vi "Adjust_VI_Properties.vi"(6 "VI refnum in":refnum<vi>, 8 "error in (no error)":errorcluster, 9 "sourceInclusion":T3, 10 "properties in":T1[](array[typedef]), 11 "AB_EXE in":refnum<class "AB_EXE.lvclass">) -> (0 "error out":errorcluster, 1 "defaultSaveLevel":u32, 2 "properties out":T1[](array[typedef]), 3 "AB_EXE out":refnum<class "AB_EXE.lvclass">)   [LabVIEW 2020, in "AB_EXE.lvclass"]
uses:
  <vilib>/AppBuilder/AB_Classes/EXE/AB_EXE.lvclass
  <vilib>/AppBuilder/AB_Source_Inclusion.ctl
  <vilib>/AppBuilder/AB_Source_Properties.ctl
  <vilib>/AppBuilder/AB_Source_Property_Type.ctl
  <vilib>/AppBuilder/AB_Classes/Application/AB_Application.lvclass
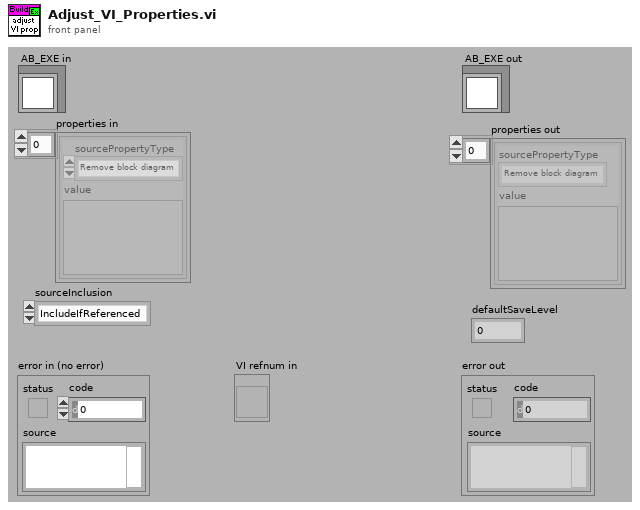
[diagram p1: front panel]
types:
  T1 = typedef "AB_Source_Properties.ctl" = cluster{"sourcePropertyType":T2, "value":variant}
  T2 = typedef "AB_Source_Property_Type.ctl" = enum16{"Remove block diagram", "Remove front panel", "Password", "Window has title bar", "Show menu bar", "Show vertical scroll bar", "Show horizontal scroll bar", "Show toolbar", "Show Abort button", "Show fp when called", "Window behavior", "Allow user to close window", "Window run-time position", "Run when opened", "Allow debugging", "Auto error handling", "Generate guard code", "Use stack variables", "Expression folding", "Integer only", "Inline subVI"}
  T3 = typedef "AB_Source_Inclusion.ctl" = enum16{"IncludeIfReferenced", "Include", "Exclude", "TopLevel"}
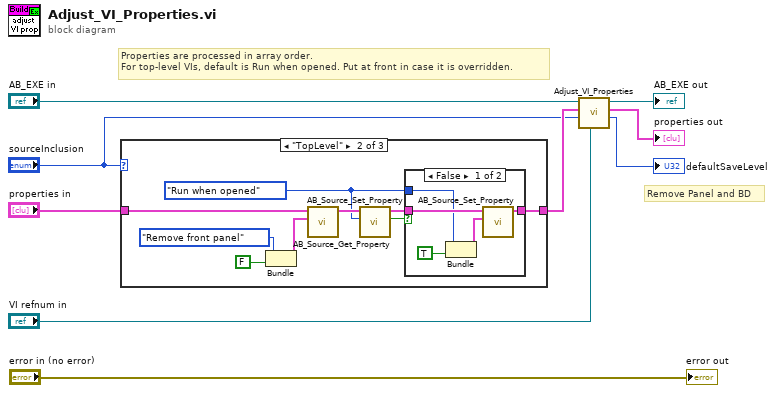
[diagram p0: block diagram]
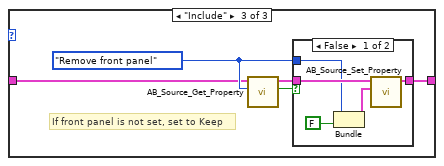
[diagram p4: hidden frame]
diagram:
  # "Remove Panel and BD"
  # "Properties are processed in array order.\nFor top-level VIs, default is Run when opened. Put at front in case it is overridden."
  n1 = case shown="\"TopLevel\"" "sourceInclusion" {
    tunnel: "properties in" -> [w10 w17 w26]
    tunnel: [w10 w12 w28] -> w3
    frame Default {
    }
    frame "TopLevel" {
      w11 = AB_Source_Property_Type."Run when opened" ("sourcePropertyType")
      n2 = Bundle("sourcePropertyType"=AB_Source_Property_Type."Remove front panel", FALSE) -> (w16:cluster{"sourcePropertyType":T2, bool})  [unwired: 1 out]
      n3 = call <vilib>:"AB_Source_Set_Property.vi"("sourceProperty"=w16, "sourceProperties in"=w17) -> ("sourceProperties out"=w15:T1[])  [unwired: 1 in, 8 out]
      n4 = call <vilib>:"AB_Source_Get_Property.vi"("type"=w11, "sourceProperties in"=w15) -> ("found"=w14:bool, "sourceProperties out"=w13:T1[])  [unwired: 1 in, 7 out]
      n5 = case shown="False" w14 {
        tunnel: w13 -> [w24 w25]
        tunnel: [w23 w25] -> w12
        tunnel: w11 -> [w21 _]
        frame False {
          n6 = Bundle("sourcePropertyType"=w21, TRUE) -> (w20:cluster{"sourcePropertyType":T2, bool})  [unwired: 1 out]
          n7 = call <vilib>:"AB_Source_Set_Property.vi"("sourceProperty"=w20, "sourceProperties in"=w24) -> ("sourceProperties out"=w23:T1[])  [unwired: 1 in, 8 out]
        }
        frame True {
        }
      }
    }
    frame "Include" {
      w27 = AB_Source_Property_Type."Remove front panel" ("sourcePropertyType")
      # "If front panel is not set, set to Keep"
      n8 = call <vilib>:"AB_Source_Get_Property.vi"("type"=w27, "sourceProperties in"=w26) -> ("found"=w30:bool, "sourceProperties out"=w29:T1[])  [unwired: 1 in, 7 out]
      n9 = case shown="False" w30 {
        tunnel: w29 -> [w35 w36]
        tunnel: [w34 w36] -> w28
        tunnel: w27 -> [w32 _]
        frame False {
          n10 = Bundle("sourcePropertyType"=w32, FALSE) -> (w31:cluster{"sourcePropertyType":T2, bool})  [unwired: 1 out]
          n11 = call <vilib>:"AB_Source_Set_Property.vi"("sourceProperty"=w31, "sourceProperties in"=w35) -> ("sourceProperties out"=w34:T1[])  [unwired: 1 in, 8 out]
        }
        frame True {
        }
      }
    }
  }
  n12 = call-parent "Adjust_VI_Properties.vi"("VI refnum in"="VI refnum in", "sourceInclusion"="sourceInclusion", "properties in"=w3, "AB_Application in"="AB_EXE in") -> ("defaultSaveLevel"=→"defaultSaveLevel":u32, "properties out"=→"properties out":T1[], "AB_Application out"=→"AB_EXE out":refnum<class "AB_EXE.lvclass">)  [unwired: 1 in, 4 out]
  "error out" <- "error in (no error)"
